vi "Build DashBoard Data.vi"(11 "Dashboard Enables":T3={"Analog Module 1"=[TRUE, TRUE, TRUE, TRUE, TRUE, TRUE, TRUE, TRUE], "Analog Module 2"=[FALSE, FALSE, FALSE, FALSE, FALSE, FALSE, FALSE, FALSE], "Digital Module 1"=TRUE, "Digital Module 2"=FALSE, "Solenoid Module"=TRUE}) -> ()   [LabVIEW 2011]
doc: "This VI builds data and sends it back to the dashboard PC program. By default it sends back the raw values for the first analog, digital, and solenoid module. Modify it to send back the data you want to view. Consider adding higher level data to the Dashboard Datatype.ctl and to this VI. Then update the Dashboard to display the data however you like.\n\nThis software is licensed. Open the labview\\readme\\WPI Robotics Library Open Source License.txt file for more information."
uses:
  DashboardEnable.ctl
  Dashboard Datatype.ctl
  <vilib>/Rock Robotics/WPI/DriverStation/WPI_DriverStationDigitalData.ctl
  Robot Global Data.vi
panel:
  out "Dashboard Data":T1
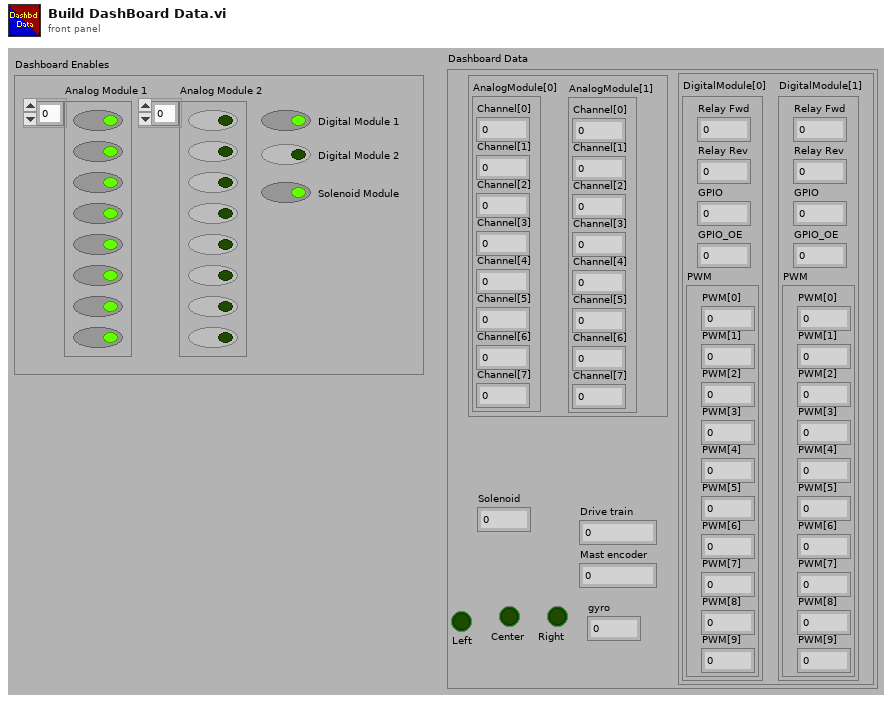
[diagram p1: front panel]
types:
  T1 = typedef "Dashboard Datatype.ctl" = cluster{cluster{"AnalogModule[0]":cluster{"Channel[0]":sgl, "Channel[1]":sgl, "Channel[2]":sgl, "Channel[3]":sgl, "Channel[4]":sgl, "Channel[5]":sgl, "Channel[6]":sgl, "Channel[7]":sgl}, "AnalogModule[1]":cluster{"Channel[0]":sgl, "Channel[1]":sgl, "Channel[2]":sgl, "Channel[3]":sgl, "Channel[4]":sgl, "Channel[5]":sgl, "Channel[6]":sgl, "Channel[7]":sgl}}, cluster{"DigitalModule[0]":T2, "DigitalModule[1]":T2}, "Solenoid":u8, "Drive train":dbl, "Mast encoder":dbl, "gyro":dbl, "Left":bool, "Center":bool, "Right":bool}
  T2 = typedef "WPI_DriverStationDigitalData.ctl" = cluster{"Relay Fwd":u8, "Relay Rev":u8, "GPIO":u16, "GPIO_OE":u16, "PWM":cluster{"PWM[0]":u8, "PWM[1]":u8, "PWM[2]":u8, "PWM[3]":u8, "PWM[4]":u8, "PWM[5]":u8, "PWM[6]":u8, "PWM[7]":u8, "PWM[8]":u8, "PWM[9]":u8}}
  T3 = typedef "DashboardEnable.ctl" = cluster{"Analog Module 1":bool[], "Analog Module 2":bool[], "Digital Module 1":bool, "Digital Module 2":bool, "Solenoid Module":bool}
  T4 = cluster{"Left":bool, "Center":bool, "Right":bool}
  T5 = cluster{"AnalogModule[0]":cluster{"Channel[0]":sgl, "Channel[1]":sgl, "Channel[2]":sgl, "Channel[3]":sgl, "Channel[4]":sgl, "Channel[5]":sgl, "Channel[6]":sgl, "Channel[7]":sgl}, "AnalogModule[1]":cluster{"Channel[0]":sgl, "Channel[1]":sgl, "Channel[2]":sgl, "Channel[3]":sgl, "Channel[4]":sgl, "Channel[5]":sgl, "Channel[6]":sgl, "Channel[7]":sgl}}
  T6 = cluster{"Channel[0]":sgl, "Channel[1]":sgl, "Channel[2]":sgl, "Channel[3]":sgl, "Channel[4]":sgl, "Channel[5]":sgl, "Channel[6]":sgl, "Channel[7]":sgl}[]
  T7 = cluster{"Channel[0]":sgl, "Channel[1]":sgl, "Channel[2]":sgl, "Channel[3]":sgl, "Channel[4]":sgl, "Channel[5]":sgl, "Channel[6]":sgl, "Channel[7]":sgl}
  T8 = cluster{"AnalogModule[0][0]":sgl, "AnalogModule[0][1]":sgl, "AnalogModule[0][2]":sgl, "AnalogModule[0][3]":sgl, "AnalogModule[0][4]":sgl, "AnalogModule[0][5]":sgl, "AnalogModule[0][6]":sgl, "AnalogModule[0][7]":sgl}
  T9 = cluster{"[0]":cluster{"Channel[0]":sgl, "Channel[1]":sgl, "Channel[2]":sgl, "Channel[3]":sgl, "Channel[4]":sgl, "Channel[5]":sgl, "Channel[6]":sgl, "Channel[7]":sgl}, "[1]":cluster{"Channel[0]":sgl, "Channel[1]":sgl, "Channel[2]":sgl, "Channel[3]":sgl, "Channel[4]":sgl, "Channel[5]":sgl, "Channel[6]":sgl, "Channel[7]":sgl}}
  T10 = cluster{"DigitalModule[0]":T2, "DigitalModule[1]":T2}
  T11 = typedef "FPGA_DIODevRef.ctl" = cluster{"DevStatus":errorcluster, "Module":T12}
  T12 = typedef "FPGA_TypedefDigitalModule.ctl" = enum16{"Digital Module 1", "Digital Module 2"}
  T13 = cluster{"[0]":u8, "[1]":u8, "[2]":u8, "[3]":u8, "[4]":u8, "[5]":u8, "[6]":u8, "[7]":u8, "[8]":u8, "[9]":u8}
  T14 = typedef "FPGA_SolenoidDevRef.ctl" = cluster{"DevStatus":errorcluster, "Module":T15}
  T15 = typedef "FPGA_TypedefSolenoidModule.ctl" = enum16{"Solenoid Module 1", "Solenoid Module 2"}
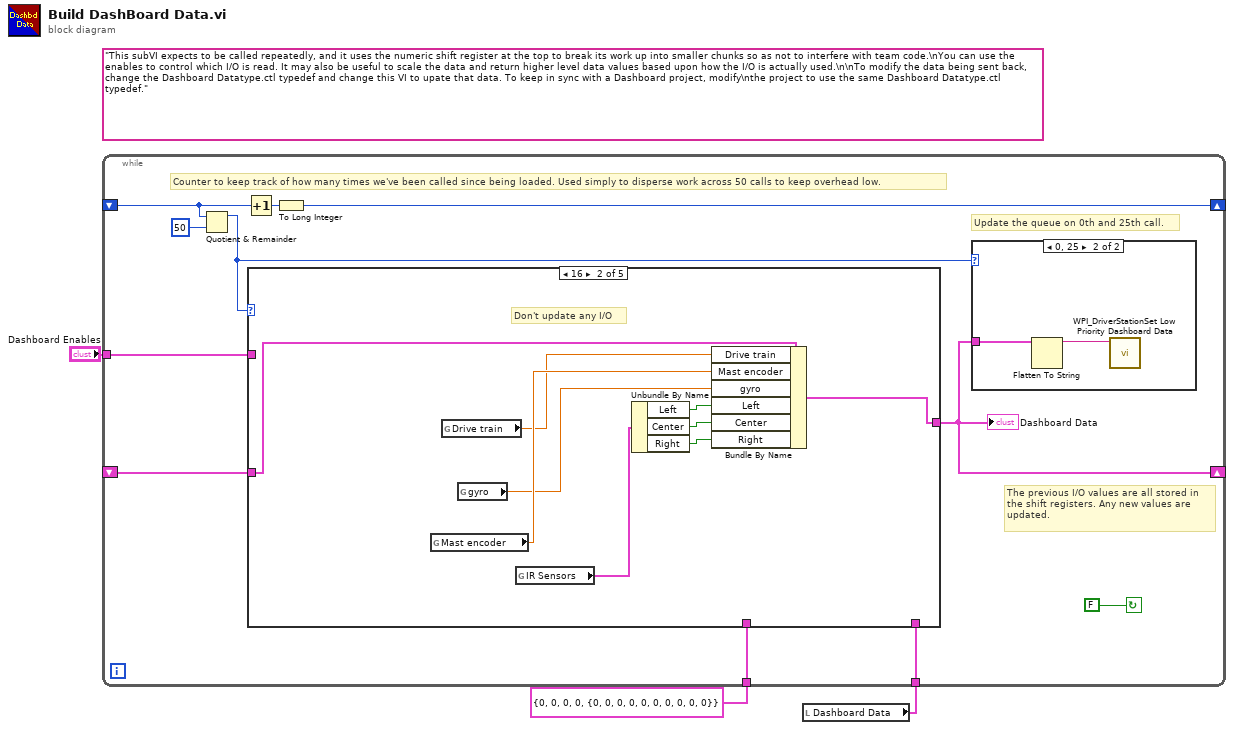
[diagram p0: block diagram]
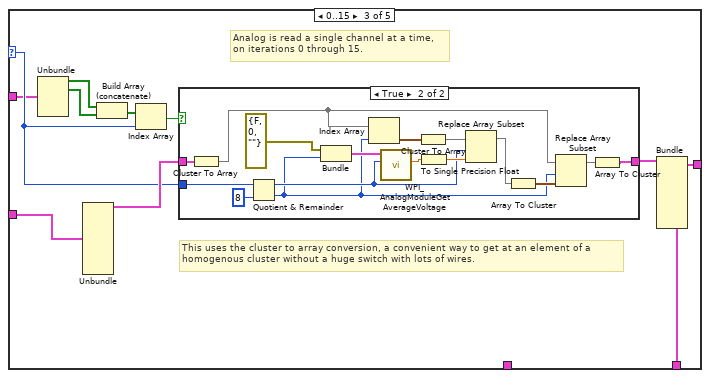
[diagram p4: hidden frame]
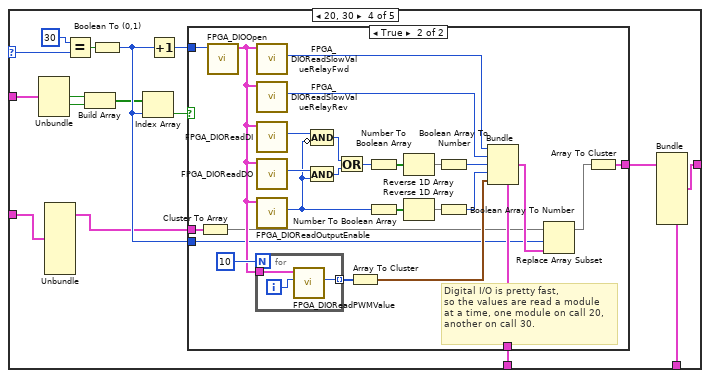
[diagram p6: hidden frame]
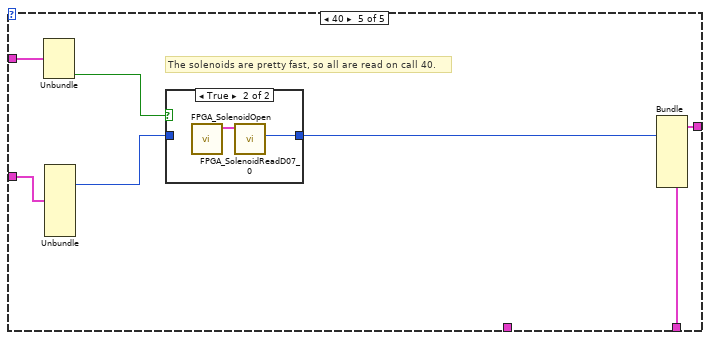
[diagram p8: hidden frame]
diagram:
  (unwired) "This subVI expects to be called repeatedly, and it uses the numeric shift register at the top to break its work up into smaller chunks so as not to interfere with team code.\nYou can use the enables to control which I/O is read. It may also be useful to scale the data and return higher level data values based upon how the I/O is actually used.\n\nTo modify the data being sent back, change the Dashboard Datatype.ctl typedef and change this VI to upate that data. To keep in sync with a Dashboard project, modify\nthe project to use the same Dashboard Datatype.ctl typedef."
  n1 = local read "Dashboard Data"() -> (w2:T1)
  n2 = while {
    shift-right: [w7] -> _
    shift-left: _ -> [w9]
    shift-right: [w4] -> _
    shift-left: _ -> [w12]
    tunnel: T2 {"Relay Fwd"=0, "Relay Rev"=0, "GPIO"=0, "GPIO_OE"=0, "PWM"={"PWM[0]"=0, "PWM[1]"=0, "PWM[2]"=0, "PWM[3]"=0, "PWM[4]"=0, "PWM[5]"=0, "PWM[6]"=0, "PWM[7]"=0, "PWM[8]"=0, "PWM[9]"=0}} ("DigitalModule[1]") -> [w11]
    tunnel: w2 -> [w6]
    tunnel: "Dashboard Enables" -> [w5]
    stop <- FALSE continue-if-true
    # "Counter to keep track of how many times we've been called since being loaded. Used simply to disperse work across 50 calls to keep overhead low."
    # "Update the queue on 0th and 25th call."
    # "The previous I/O values are all stored in\nthe shift registers. Any new values are\nupdated."
    n3 = Quotient & Remainder(x=w9, y=50) -> (x-y*floor(x/y)=w8:i32)  [unwired: 1 out]
    n4 = Increment(x=w9) -> (x+1=w14:i32)
    n5 = case shown="16" w8 {
      selector: w8 -> [_ _ w32 w64 _]
      tunnel: [w17 w25 w28 w55 w104] -> w4
      tunnel: w12 -> [w17 w26 w27 w57 w106]
      tunnel: w11 -> [_ _ _ w70 _]
      tunnel: w6 -> [_ _ w34 w56 w103]
      tunnel: w5 -> [_ _ w31 w62 w107]
      frame Default {
        # "Don't update any I/O"
      }
      frame 16 {
        # "Don't update any I/O"
        n6 = global read "Robot Global Data.vi" "Mast encoder"() -> (w24:dbl)
        n7 = global read "Robot Global Data.vi" "Drive train"() -> (w22:dbl)
        n8 = global read "Robot Global Data.vi" "gyro"() -> (w23:dbl)
        n9 = global read "Robot Global Data.vi" "IR Sensors"() -> (w21:T4)
        n10 = Unbundle By Name(w21) -> ("Left"=w20:bool, "Center"=w19:bool, "Right"=w18:bool)
        n11 = Bundle By Name(cluster=w26, "Drive train"=w22, "Mast encoder"=w24, "gyro"=w23, "Left"=w20, "Center"=w19, "Right"=w18) -> (w25:T1)
      }
      frame 0..15 {
        # "This uses the cluster to array conversion, a convenient way to get at an element of a\nhomogenous cluster without a huge switch with lots of wires."
        # "Analog is read a single channel at a time,\non iterations 0 through 15."
        n12 = Unbundle(w31) -> ("Analog Module 1"=w30:bool[], "Analog Module 2"=w29:bool[])  [unwired: 3 out]
        n13 = Unbundle(w27) -> (w33:T5)  [unwired: 8 out]
        n14 = Build Array (concatenate)(w30, w29) -> (w36:bool[])
        n15 = Index Array(array=w36, index=w32) -> (element=w37:bool)
        n16 = case shown="True" w37 {
          tunnel: w32 -> [_ w45]
          tunnel: [w38 w42] -> w35
          tunnel: w33 -> [w38 w41]
          frame False {
          }
          frame True {
            n17 = Cluster To Array(cluster=w41) -> (array=w40:T6)
            n18 = Quotient & Remainder(x=w45, y=8) -> (x-y*floor(x/y)=w44:i32, floor(x/y)=w39:i32)
            n19 = Bundle("DevStatus"=errorcluster {"status"=FALSE, "code"=0, "source"=""}, w39) -> (w53:cluster{"DevStatus":errorcluster, i32})  [unwired: 1 out]
            n20 = Index Array(array=w40, index=w39) -> (element=w47:T7)
            n21 = call <vilib>:"WPI_AnalogModuleGetAverageVoltage.vi"("Channel"=w44, "AnalogModuleDevStatus"=w53) -> ("Average Voltage"=w50:dbl)  [unwired: 1 in, 8 out]
            n22 = Cluster To Array(cluster=w47) -> (array=w46:sgl[])
            n23 = To Single Precision Float(number=w50) -> (single precision float=w49:sgl)
            n24 = Replace Array Subset(array=w46, new element=w49, index=w44) -> (w48:sgl[])
            n25 = Array To Cluster(array=w48) -> (cluster=w52:T8)
            n26 = Replace Array Subset(array=w40, new element=w52, index=w39) -> (w43:T6)
            n27 = Array To Cluster(array=w43) -> (cluster=w42:T9)
          }
        }
        n28 = Bundle(cluster=w34, w35) -> (w28:T1)  [unwired: 8 out]
      }
      frame 20, 30 {
        n29 = Unbundle(w62) -> ("Digital Module 1"=w61:bool, "Digital Module 2"=w60:bool)  [unwired: 3 out]
        n30 = Unbundle(w57) -> (w59:T10)  [unwired: 8 out]
        n31 = Equal?(x=30, y=w64) -> (x = y?=w68:bool)
        n32 = Build Array(w61, w60) -> (w63:bool[])
        n33 = Boolean To (0,1)(Boolean=w68) -> (0, 1=w66:i16)
        n34 = Index Array(array=w63, index=w66) -> (element=w65:bool)
        n35 = Increment(x=w66) -> (x+1=w67:i16)
        n36 = case shown="True" w65 {
          tunnel: w70 -> [_ w79]
          tunnel: [w71 w72] -> w58
          tunnel: w67 -> [_ w77]
          tunnel: w66 -> [_ w76]
          tunnel: w59 -> [w71 w75]
          frame False {
          }
          frame True {
            # "Digital I/O is pretty fast,\nso the values are read a module\nat a time, one module on call 20,\nanother on call 30."
            n37 = Cluster To Array(cluster=w75) -> (array=w74:T2[])
            n38 = call <vilib>:"FPGA_DIOOpen.vi"("Module (Module 1)"=w77) -> ("DIODeviceRef"=w95:T11)  [unwired: 1 in, 9 out]
            n39 = for {
              N: 10 -> [_]
              tunnel: w95 -> [w100]
              tunnel: [w98] -> w96 mode=indexing
              i -> [w99]
              n40 = call <vilib>:"FPGA_DIOReadPWMValue.vi"("PWMChannel"=w99, "DIODeviceRef In"=w100) -> ("PWMValue"=w98:u8)  [unwired: 1 in, 8 out]
            }
            n41 = call <vilib>:"FPGA_DIOReadSlowValueRelayFwd.vi"("DIODeviceRef In"=w95) -> ("Relay Forward"=w88:u8)  [unwired: 1 in, 9 out]
            n42 = call <vilib>:"FPGA_DIOReadSlowValueRelayRev.vi"("DIODeviceRef In"=w95) -> ("Relay Reverse"=w89:u8)  [unwired: 1 in, 9 out]
            n43 = call <vilib>:"FPGA_DIOReadDI.vi"("DIODeviceRef In"=w95) -> ("DI"=w93:u16)  [unwired: 1 in, 9 out]
            n44 = call <vilib>:"FPGA_DIOReadDO.vi"("DIODeviceRef In"=w95) -> ("DO"=w92:u16)  [unwired: 1 in, 9 out]
            n45 = call <vilib>:"FPGA_DIOReadOutputEnable.vi"("DIODeviceRef In"=w95) -> ("OutputEnable"=w83:u16)  [unwired: 1 in, 9 out]
            n46 = And(x=w92, y=w83) -> (x .and. y?=w91:u16)
            n47 = Compound Arithmetic op=AND(w93, invert w83) -> (w90:u16)
            n48 = Or(x=w90, y=w91) -> (x .or. y?=w81:u16)
            n49 = Array To Cluster(array=w96) -> (cluster=w94:T13)
            n50 = Number To Boolean Array(number=w81) -> (Boolean array=w86:bool[])
            n51 = Number To Boolean Array(number=w83) -> (Boolean array=w85:bool[])
            n52 = Reverse 1D Array(array=w86) -> (reversed array=w87:bool[])
            n53 = Reverse 1D Array(array=w85) -> (reversed array=w84:bool[])
            n54 = Boolean Array To Number(Boolean array=w87) -> (number=w80:u32)
            n55 = Boolean Array To Number(Boolean array=w84) -> (number=w82:u32)
            n56 = Bundle(cluster=w79, "Relay Fwd"=w88, "Relay Rev"=w89, "GPIO"=w80, "GPIO_OE"=w82, "PWM"=w94) -> (w78:T2)
            n57 = Replace Array Subset(array=w74, new element=w78, index=w76) -> (w73:T2[])
            n58 = Array To Cluster(array=w73) -> (cluster=w72:cluster{"[0]":T2, "[1]":T2})
          }
        }
        n59 = Bundle(cluster=w56, w58) -> (w55:T1)  [unwired: 8 out]
      }
      frame 40 {
        # "The solenoids are pretty fast, so all are read on call 40."
        n60 = Unbundle(w107) -> ("Solenoid Module"=w101:bool)  [unwired: 4 out]
        n61 = Unbundle(w106) -> ("Solenoid"=w105:u8)  [unwired: 8 out]
        n62 = case shown="True" w101 {
          tunnel: [w108 w109] -> w102
          tunnel: w105 -> [w108 _]
          frame False {
          }
          frame True {
            n63 = call <vilib>:"FPGA_SolenoidOpen.vi"() -> ("SolenoidDevRef"=w110:T14)  [unwired: 2 in, 9 out]
            n64 = call <vilib>:"FPGA_SolenoidReadD07_0.vi"("SolenoidDevRef"=w110) -> ("DO7:0"=w109:u8)  [unwired: 1 in, 9 out]
          }
        }
        n65 = Bundle(cluster=w103, "Solenoid"=w102) -> (w104:T1)  [unwired: 8 out]
      }
    }
    "Dashboard Data" <- w4
    n66 = To Long Integer(number=w14) -> (32bit integer=w7:i32)
    n67 = case shown="0, 25" w8 {
      tunnel: w4 -> [_ w16]
      frame Default {
      }
      frame 0, 25 {
        n68 = Flatten To String(anything=w16) -> (data string=w15:string)  [unwired: 1 in, 4 out]
        n69 = call <vilib>:"WPI_DriverStationSet Low Priority Dashboard Data.vi"("User Data"=w15) -> ()  [unwired: 1 in, 10 out]
      }
    }
  }
